vi "View A-Scan.vi"(10 "A-Scan Processed":sgl[](graph)=[-26.210978, -0.31578374, -1.8610598, -13.492583, -27.979498, -5.7245455, -0.3292389, -4.510563, -14.818077, -30.297182, -19.535238, -8.432641, -0.8121514, -1.7452242, -11.954155, -16.504982, -5.743655, -5.071388, -12.874917, -27.469084, -28.696384, -23.557272, -18.030994, -15.969668, -11.015175, -11.5916395, -19.863699, -26.249102, -22.386854, -29.339754, -25.127794, -33.261314, -28.425385, -31.03366, -23.45998, -24.344952, -31.405022, -32.837296, -28.08223, -25.55752, -25.279045, -26.942255, -26.625408, -24.167088, -27.910465, -29.274937, -22.219278, -20.05723, -26.108677, -22.097414, -27.75035, -32.056778, -29.910599, -24.903984, -27.671215, -29.608793, -44.94435, -32.444386, -36.56743, -24.9354, -26.683678, -23.9393, -25.238876, -35.807644, -28.46127, -33.92609, -23.394852, -20.960835, -19.181705, -18.781902, -22.780018, -31.818577, -28.909134, -22.674618, -25.622366, -31.60658, -29.545992, -34.63347, -27.351624, -45.00616, -30.52248, -34.17556, -26.224926, -28.119835, -25.108356, -32.589897, -21.198568, -21.048626, -24.815128, -20.277594, -22.449446, -22.564396, -23.654078, -19.366909, -25.552483, -17.816277, -18.52091, -25.534723, -25.30511, -21.510155, -21.73051, -23.231468, -23.07098, -25.038015, -21.5863, -38.30931, -27.069336, -29.471285, -23.319408, -23.01601, -24.3645, -32.88109, -23.353159, -25.882452, -28.715004, -34.466026, -34.025963, -35.122337, -22.841404, -22.532616, -12.578817, -11.619661, -17.050789, -25.473412, -30.49468, -31.098743, -41.366486, -28.964567, -38.44023, -26.351032, -21.317728, -21.813507, -23.792786, -20.529749, -20.11974, -23.277401, -27.823189, -26.973354, -24.241344, -24.333897, -26.06728, -53.132034, -32.367374, -31.709272, -29.559715, -35.48095, -40.987263, -30.28252, -28.209124, -29.503412, -27.401718, -27.646305, -22.93663, -22.070507, -33.09205, -34.82585, -27.275171, -32.58675, -29.522762, -22.635445, -23.142614, -27.973444, -26.65776, -27.490786, -39.08202, -23.444656, -22.362215, -22.415667, -33.80705, -28.281424, -26.454248, -37.24972, -43.585503, -27.439075, -27.784927, -27.602098, -32.125473, -35.726906, -36.536613, -31.075264, -38.49138, -27.625084, -26.77308, -27.488235, -29.514954, -22.231047, -29.748785, -33.403545, -27.761621, -26.688044, -25.825941, -35.921432, -43.165215, -26.127644, -26.853542, -24.654018, -22.703587, -27.379139, -35.317154, -24.985218, -20.411322, -22.853783, -30.926537, -30.707005, -31.797073, -31.337273, -26.2733, -23.047895, -22.52106, -27.7406, -27.451904, -33.804142, -27.606064, -25.81736, -27.720068, -36.016445, -27.700396, -27.664001, -30.901567, -27.07572, -32.00824, -26.91952, -23.52076, -23.271412, -25.111042, -34.587776, -32.977566, -25.886318, -24.229359, -26.734869, -32.142445, -26.288021, -30.677977, -52.17713, -24.04543, -22.249277, -34.459236, -30.383837, -32.543636, -32.750458, -26.37726, -23.7031, -27.623089, -32.123077, -40.254158, -23.576668, -24.094315, -30.320057, -31.964115, -29.275007, -33.622116, -30.901989, -25.8515, -22.568684, -24.535221, -25.86589, -37.747265, -31.16762, -36.97809, -34.62544, -29.410555, -25.7421, -24.113754, -24.21185, -26.27621, -28.80848, -33.13751, -29.363487, -31.258715, -24.950201, -27.174103, -22.409803, -22.727638, -30.952318, -31.949465, -33.96205, -32.321663, -41.727978, -26.914566, -23.141737, -22.170698, -20.978714, -27.677824, -24.802229, -20.999434, -25.072222, -28.95887, -32.70508, -28.58545, -27.07776, -24.924133, -25.208416, -28.979347, -25.955524, -32.08485, -28.693113, -29.154903, -37.858196, -39.133152, -36.21201, -25.883911, -23.183058, -25.838087, -26.123013, -29.354885, -27.11465, -24.470499, -27.968615, -23.639149, -23.14795, -26.119194, -35.968136, -28.441235, -23.77411, -23.665869, -31.111137, -31.179775, -28.989357, -27.464413, -32.31834, -26.286488, -27.108946, -29.648035, -27.614647, -36.93215, -32.280243, -29.210852, -25.338709, -27.051355, -25.309155, -23.086699, -31.160858, -28.991549, -27.485672, -27.540636, -21.71913, -26.28127, -31.117641, -23.571243, -22.516005, -29.04525, -32.098057, -25.547585, -42.95463, -31.956524, -22.141758, -17.952759, -19.610708, -23.644444, -27.758587, -25.057549, -26.134052, -25.293467, -29.953926, -29.844152, -23.126877, -26.776941, -33.989, -28.728153, -32.912956, -23.412436, -26.758936, -22.57225, -21.015762, -29.183378, -25.705784, -23.323528, -23.375137, -23.703573, -35.110134, -26.101551, -24.078419, -26.154135, -22.656559, -21.120544, -27.295572, -24.547276, -24.689686, -35.097187, -19.975447, -20.70405, -30.063946, -27.709393, -24.640957, -32.71785, -28.640612, -20.957756, -20.722157, -26.627188, -31.318886, -29.09002, -27.642347, -24.033022, -32.032455, -26.147396, -32.72879, -33.134163, -25.682604, -26.329826, -34.172707, -45.549637, -32.19201, -28.775599, -27.236197, -36.347317, -35.575523, -26.131685, -28.427603, -31.673988, -36.608932, -34.141914, -42.357056, -29.318504, -28.417885, -32.167183, -34.500694, -27.596508, -31.125277, -26.832617, -21.614109, -22.663319, -29.111574, -24.030752, -22.409107, -31.82102, -32.892212, -32.415745, -26.740353, -25.385103, -26.80175, -24.186478, -22.655315, -22.39489, -21.797451, -20.889229, -23.851068, -24.81073, -21.483337, -21.090714, -26.381187, -26.369854, -24.48166, -23.760208, -23.644342, -25.481583, -21.709759, -20.336998, -22.738392, -24.181318, -23.530704, -24.073698, -25.371855, -29.36827, -33.906986, -22.88837, -22.117483, -34.872936, -31.19501, -25.523607, -21.588385, -20.013102, -18.8254, -18.81281, -26.45252, -31.17826, -31.253874, -27.593842, -32.520233, -24.856508, -23.329897, -29.87441, -37.53676, -23.516674, -20.780876, -25.053402, -25.033222, -23.65327, -23.898222, -19.479591, -22.383928, -31.456697, -31.780369, -23.594852, -26.903454, -26.312883, -47.82139, -24.327026, -24.945843, -27.786072, -20.467207, -25.291618, -24.066692, -36.908745, -23.990826, -22.015648, -21.728424, -24.255674, -25.284016, -17.604519, -21.369007, -24.234962, -21.949186, -23.958088, -23.777592, -17.950075, -22.514679, -30.692993, -32.666252, -28.321722, -26.032763, -31.239384, -23.781271, -25.228098, -24.143929, -24.327179, -21.55861, -22.293808, -40.871967, -31.49052, -26.345123, -31.653671, -38.96815, -31.11382, -30.299416, -34.112003, -29.309956, -19.669268, -20.856876, -25.5818, -25.964798, -23.235428, -20.267351, -21.306042, -25.324953, -32.886566, -33.848198, -30.231703, -19.943031, -20.70887, -31.18996, -38.037865, -25.804028, -23.056585, -26.322596, -38.74378, -28.29768, -27.166054, -27.325365, -22.84835, -23.460272, -23.510675, -25.210625, -29.019207, -29.465004, -34.738686, -28.07248, -29.004747, -37.84001, -30.637262, -30.132875, -24.175072, -25.127258, -26.92854, -28.183363, -22.317673, -29.53536, -32.943462, -22.5015, -17.434628, -17.622349, -21.835793, -21.983576, -21.254726, -24.232197, -30.984581, -35.853207, -32.10312, -19.321465, -17.624142, -20.444664, -21.004726, -22.67358, -25.06542, -21.320122, -23.435019, -27.823555, -26.044563, -24.597794, -22.637848, -24.535957, -34.368435, -24.400473, -20.907734, -25.545467, -35.642853, -26.396896, -25.6619, -25.823061, -20.670412, -20.21106, -29.578287, -29.226358, -30.222311, -27.00819, -28.136663, -29.100351, -28.457932, -24.669703, -25.028812, -18.786524, -19.427868, -25.43777, -21.199684, -15.573761, -1.0208147, 7.6145773, 10.022359, 7.7157907, 6.070616, 9.813012, 15.933785, 22.136951, 25.04485, 23.8101, 16.993906, 3.8796186, 15.961233, 16.285875, 13.045634, 7.2316785, 2.657391, -4.7237477, -6.347074, -5.0806813, -11.554905, -26.610163, -9.1125765, -11.753917, -10.766447, -12.167433, -17.402613, -9.076464, -10.4888525, -20.842134, -13.619364, -16.773762, -19.546986, -23.723976, -25.914572, -28.425293, -18.009684, -15.721116, -19.651096, -22.298372, -26.993717, -21.207827, -33.86458, -16.998291, -19.768642, -22.319141, -18.725727, -20.68567, -23.248938, -33.058094, -35.201458, -30.761806, -26.134024, -40.351723, -17.83051, -14.775904, -20.180481, -26.82964, -22.300451, -23.828773, -22.818367, -23.048168, -26.578943, -26.982422, -30.778564, -32.837204, -29.521778, -31.278343, -35.43119, -36.43036, -31.21062, -26.882355, -25.316109, -30.444912], 11 "A-Scan (Raw)":u16[](graph)=[33360, 31728, 32832, 32768, 32272, 32560, 32976, 32608, 33136, 31744, 33296, 31472, 32848, 33264, 31968, 33120, 32272, 32608, 32944, 32112, 33456, 32016, 33584, 31952, 33488, 31552, 33632, 33344, 33360, 32128, 32368, 33232, 31824, 33280, 31632, 34576, 31136, 33456, 31360, 33344, 32208, 32848, 32800, 31920, 34288, 31168, 33520, 31408, 33488, 31760, 33264, 32544, 32352, 33280, 31904, 33696, 31808, 33776, 32256, 33456, 32096, 32864, 32800, 32304, 33408, 31952, 33840, 31568, 33584, 31888, 33424, 32448, 32592, 33008, 32032, 33584, 31856, 33872, 32112, 33328, 32096, 32704, 32752, 32368, 33632, 32176, 33456, 31776, 33456, 31952, 33184, 32256, 32640, 32848, 32096, 33408, 31808, 33552, 32464, 34304, 31952, 32800, 32576, 32224, 33216, 32144, 33472, 31936, 33920, 31920, 33168, 33216, 32448, 32800, 32128, 33424, 31760, 33408, 31904, 33328, 32208, 32960, 32912, 32368, 33104, 32016, 33328, 31808, 33856, 31888, 33248, 32592, 32928, 32896, 32464, 33456, 32464, 33232, 31968, 33264, 32160, 33120, 32672, 33008, 32864, 32208, 33232, 31968, 33264, 31744, 33200, 32160, 32864, 32752, 32496, 33280, 32256, 33408, 32176, 33488, 32096, 32976, 32320, 32720, 32976, 32288, 33232, 31888, 33568, 31776, 33408, 32096, 32976, 32480, 32656, 33168, 32240, 33408, 31936, 33552, 32048, 33312, 32080, 32768, 32736, 32320, 33328, 32128, 33632, 31872, 33584, 31632, 33296, 32048, 32688, 32912, 32224, 33392, 31600, 33920, 31600, 33952, 31728, 33264, 32304, 32512, 33008, 31872, 33840, 31408, 34176, 31520, 33936, 31776, 33376, 32576, 32240, 33376, 31440, 34064, 31136, 34416, 31280, 34016, 31936, 33232, 32928, 32096, 33584, 31200, 34288, 30864, 34384, 31280, 33952, 32000, 32800, 33088, 31600, 33936, 30752, 34480, 30608, 34304, 31216, 33504, 32256, 32464, 33456, 31120, 34352, 30464, 34704, 30448, 34496, 31232, 33488, 32480, 32144, 33952, 30944, 34608, 30432, 34736, 30752, 34176, 31760, 33152, 33232, 31872, 34368, 30672, 35056, 30480, 34656, 30976, 33840, 32352, 32512, 33808, 31184, 34912, 30496, 35056, 30512, 34432, 31520, 33248, 32864, 31744, 34224, 30736, 35184, 30240, 34928, 30704, 33968, 31952, 32624, 33744, 31152, 34848, 30480, 35344, 30416, 34816, 31216, 33488, 32640, 32048, 34000, 30800, 35040, 30304, 35280, 30704, 34560, 31872, 32992, 33232, 31632, 34400, 30560, 35280, 30352, 35088, 31120, 33888, 32544, 32608, 33696, 31248, 34832, 30576, 35152, 30640, 34800, 31376, 33552, 32784, 32208, 33952, 30992, 34608, 30608, 34704, 30864, 34064, 31888, 32992, 33264, 31632, 34080, 30752, 34416, 30608, 34144, 31312, 33568, 32432, 32144, 33488, 31328, 34160, 30752, 34272, 30880, 33904, 31744, 32960, 32912, 31984, 33776, 31184, 34192, 31008, 34016, 31360, 33456, 32096, 32752, 33328, 31776, 34096, 31312, 34160, 31296, 33872, 31840, 33152, 32688, 32176, 33696, 31600, 34208, 31408, 34112, 31504, 33520, 32208, 32848, 32880, 31904, 33792, 31440, 34096, 31456, 33952, 31776, 33296, 32496, 32464, 33200, 31664, 33888, 31152, 34080, 31344, 33808, 31904, 33024, 32768, 32096, 33488, 31328, 34016, 31104, 34096, 31408, 33712, 32160, 32640, 33120, 31744, 33744, 31264, 34176, 30992, 34000, 31600, 33296, 32560, 32384, 33440, 31344, 34096, 31056, 34272, 31136, 34000, 31888, 33056, 32880, 31888, 34016, 30992, 34480, 30560, 34448, 30976, 33648, 32224, 32448, 33456, 31312, 34336, 30432, 34800, 30240, 34528, 31040, 33376, 32432, 31776, 34048, 30528, 35088, 29744, 35376, 29936, 34672, 31072, 33152, 33168, 31200, 34624, 29968, 35760, 29344, 35600, 29904, 34336, 31520, 32720, 33472, 30896, 35312, 29472, 36144, 29344, 35536, 30320, 34240, 32048, 32144, 34496, 30144, 35984, 29152, 36432, 29392, 35456, 30864, 33664, 33008, 31200, 35056, 29648, 36464, 28912, 36368, 29648, 35216, 31408, 32864, 34000, 30336, 35824, 28832, 36672, 28784, 36304, 29968, 34576, 32336, 31712, 34800, 29776, 36512, 28592, 36848, 29104, 35808, 30608, 33808, 33296, 31264, 35344, 29136, 36752, 28688, 36752, 29376, 35472, 31344, 33008, 34128, 30544, 36032, 28976, 36848, 28816, 36528, 30112, 34720, 32080, 32496, 34512, 30112, 36288, 28640, 36880, 28880, 35792, 30448, 34048, 32704, 31728, 34960, 29728, 36336, 28880, 36544, 29152, 35344, 31248, 33360, 33248, 30960, 35088, 29488, 36128, 29024, 36048, 29824, 34672, 31632, 32800, 33520, 30800, 35312, 29504, 35968, 29264, 35552, 30272, 34288, 32080, 32288, 33920, 30752, 35344, 29696, 35744, 29840, 35120, 30896, 33808, 32576, 32256, 34208, 30928, 35088, 30192, 35440, 30384, 34800, 31328, 33712, 32784, 31984, 34208, 30880, 35008, 30496, 35168, 30768, 34544, 31680, 33200, 32976, 31984, 34048, 31120, 34784, 30816, 34720, 31216, 33984, 32096, 32976, 33136, 31888, 34064, 31152, 34640, 31024, 34496, 31264, 33920, 32256, 32688, 33296, 31728, 34128, 31264, 34384, 31120, 34208, 31488, 33488, 32368, 32528, 33248, 31584, 33888, 31168, 34192, 31200, 33936, 31616, 33248, 32416, 32256, 33296, 31376, 34016, 30992, 34096, 31168, 33648, 31680, 33088, 32608, 31952, 33312, 31392, 33888, 31136, 33888, 31296, 33392, 32048, 32656, 32912, 31808, 33488, 31248, 33904, 31328, 33648, 31728, 33168, 32528, 32336, 33440, 31584, 33936, 31408, 34112, 31568, 33680, 32368, 33024, 33120, 32176, 33712, 31648, 34176, 31536, 33936, 31952, 33328, 32768, 32576, 33504, 32016, 34256, 31552, 34304, 31664, 33824, 32368, 33120, 33232, 32336, 34064, 31568, 34480, 31504, 34208, 31968, 33584, 32640, 32656, 33648, 31776, 34352, 31312, 34528, 31424, 34144, 32064, 33328, 33328, 32144, 34160, 31344, 34608, 31184, 34512, 31408, 33936, 32416, 32928, 33456, 31952, 34368, 31216, 34736, 31184, 34528, 31696, 33648, 33008, 32512, 33904, 31488, 34624, 30960, 34768, 31200, 34400, 31872, 33120, 33104, 31952, 34240, 31024, 34928, 30752, 34848, 31136, 34256, 32240, 32928, 33360, 31824, 34432, 30928, 35056, 30656, 34992, 31200, 34144, 32224, 32768, 33824, 31424, 34816, 30656, 35232, 30608, 34944, 31232, 33936, 32608, 32672, 33904, 31264, 34928, 30496, 35296, 30512, 34960, 31280, 33936, 32480, 32624, 33872, 31344, 34976, 30528, 35312, 30544, 34928, 31216, 33920, 32512, 32496, 33952, 31184, 34976, 30496, 35168, 30560, 34944, 31200, 33712, 32864, 32304, 34080, 31248, 35040, 30512, 35328, 30736, 34880, 31312, 33776, 32784, 32512, 33824, 31216, 35024, 30560, 35344, 30576, 34880, 31232, 33872, 32592, 32544, 34144, 31232, 35040, 30592, 35200, 30640, 34688, 31392, 33504, 32816, 32256, 33968, 31344, 34896, 30624, 35136, 30816, 34512, 31648, 33568, 32672, 32352, 33824, 30960, 34704, 30512, 34960, 30736, 34528, 31488, 33216, 32448, 32048, 33808, 30912, 34528, 30432, 34752, 30672, 34224, 31376, 33344, 32544, 32272, 33648, 31008, 34192, 30608, 34400, 30816, 33920, 31488, 33184, 32544, 32096, 33536, 31376, 34128, 30992, 34176, 31280, 33744, 31984, 32944, 32768, 32272, 33616, 31696, 34080, 31600, 34096, 31824, 33824, 32400, 32928, 33056, 32240, 33600, 31872, 34032, 31872, 34096, 32144, 33680, 32752, 33088, 33344, 32544, 33712, 32208, 33984, 32064, 33904, 32656, 33456, 33072, 32992, 33552, 32608, 33824, 32464, 34000, 32336, 33632, 32752, 33312, 33104, 32832, 33552, 32528, 33840, 32336, 33776, 32272, 33648, 32784, 33152, 32976, 32656, 33456, 32304, 33488, 32256, 33568, 32352, 33440, 32864, 32976, 33120, 32544, 33376, 32208, 33392, 32112, 33376, 32320, 32944, 32656, 32736, 32960, 32352, 33232, 32320, 33328, 32272, 33200, 32400, 32912, 32704, 32544, 33088, 32144, 33328, 32160, 33312, 32352, 33088, 32688, 32848, 33168, 32416, 33424, 32176, 33568, 32112, 33296, 32384, 33040, 32880, 32640, 33344, 32368, 33744, 32192, 33904, 32288, 33600, 32720, 33184, 32832, 32640, 33392, 32160, 33872, 31952, 34016, 32080, 33776, 32768, 33232, 33104, 32688, 33520, 31952, 33872, 31744, 33824, 31952, 33456, 32336, 33008, 33008, 32432, 33648, 31760, 34032, 31616, 33888, 31872, 33344, 32176, 32800, 32912, 32112, 33552, 31520, 33968, 31376, 33872, 31808, 33488, 32368, 32640, 32928, 31952, 33456, 31312, 33952, 31024, 33760, 31520, 33264, 32240, 32512, 33120, 31856, 33776, 31136, 34112, 31056, 33888, 31584, 33248, 32304, 32432, 33104, 31728, 33856, 31008, 34352, 31136, 34176, 31504, 33632, 32336, 32512, 33152, 31632, 33872, 30992, 34256, 31024, 34144, 31360, 33600, 32336, 32800, 33312, 31872, 33968, 31088, 34304, 31136, 34192, 31408, 33712, 32256, 32656, 33184, 31872, 33952, 31312, 34240, 31104, 34176, 31536, 33472, 32096, 32496, 32992, 31808, 33568, 31376, 34016, 31136, 34144, 31536, 33536, 32304, 32880, 33152, 32128, 33648, 31600, 33888, 31360, 33776, 31760, 33264, 32304, 32592, 33136, 32080, 33792, 31744, 33968, 31696, 33920, 32032, 33456, 32576, 32736, 33120, 32144, 33616, 31744, 33856, 31808, 33792, 32064, 33552, 32800, 32992, 33200, 32432, 33616, 31936, 33776, 31936, 33680, 32096, 33280, 32752, 32816, 33312, 32512, 33616, 32224, 33648, 32224, 33488, 32432, 33056, 32768, 32624, 33184, 32256, 33536, 32000, 33648, 32064, 33360, 32352, 33024, 32800, 32688, 33056, 32224, 33376, 31824, 33568, 31952, 33280, 32240, 32864, 32688, 32544, 33088, 32208, 33248, 31984, 33392, 31904, 33232, 32080, 32784, 32624, 32448, 32752, 32256, 33152, 32048, 33344, 31984, 33328, 32304, 32960, 32848, 32656, 32944, 32256, 33136, 32208, 33296, 32128, 33104, 32352, 32832, 32672, 32656, 33168, 32464, 33312, 32528, 33264, 32576, 33184, 32576, 32832, 32848, 32608, 33152, 32368, 33168, 32512, 33040, 32784, 33040, 32992, 32800, 33008, 32512, 33248, 32224, 33312, 32464, 33120, 32688, 32800, 32960, 32528, 33104, 32448, 33248, 32304, 33296, 32368, 33072, 32880, 32592, 33328, 32208, 33296, 32176, 33136, 32032, 33184, 32160, 32880, 32720, 32432, 33008, 31920, 33328, 31952, 33360, 31888, 33168, 31968, 32800, 32304, 32144, 32976, 31552, 33168, 31328, 33200, 31728, 32912, 32064, 32848, 32464, 32448, 33120, 31904, 33344, 31568, 33360, 31712, 33008, 32128, 32608, 32816]) -> ()   [LabVIEW 2015, in "Processing.lvclass"]
uses:
  Processing.lvclass
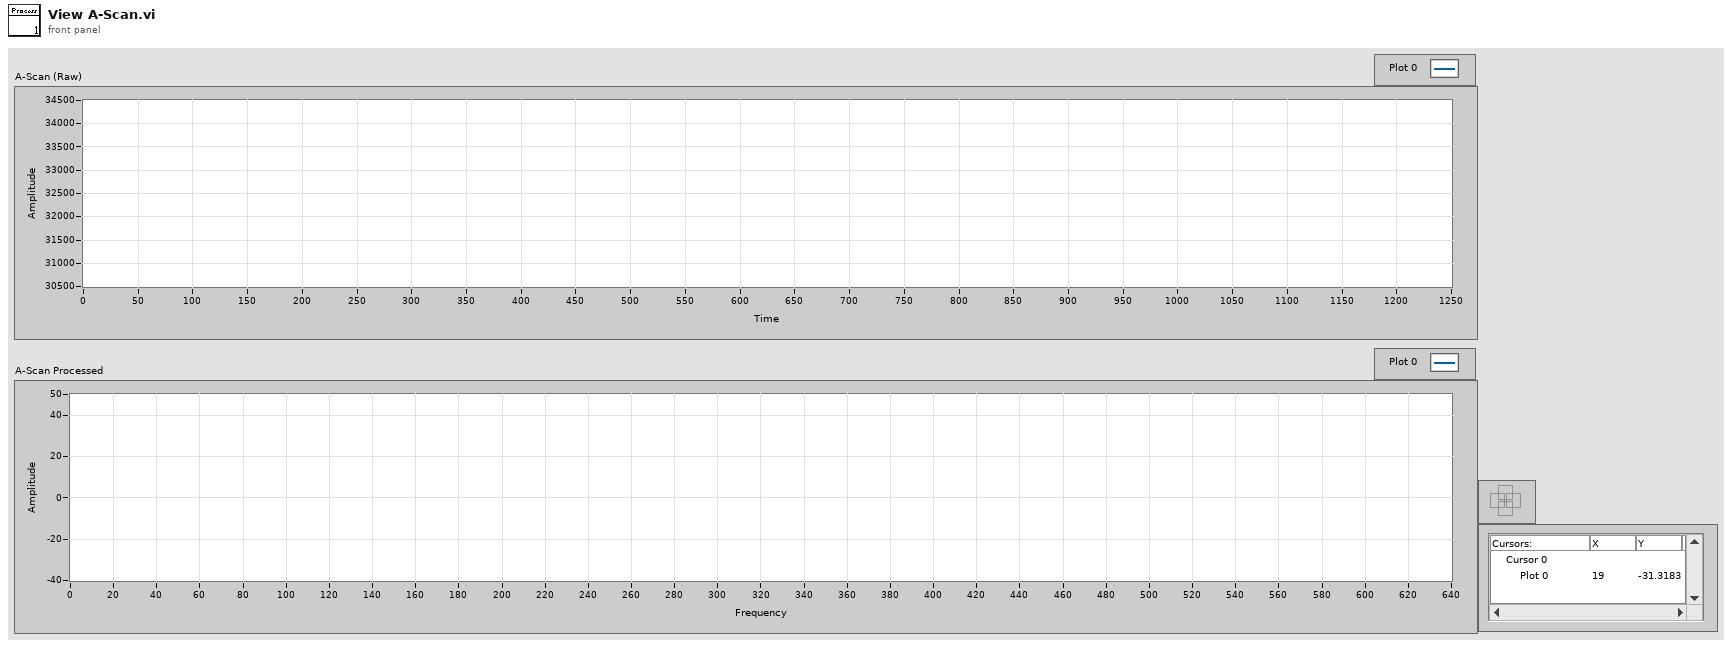
[diagram p1: front panel]
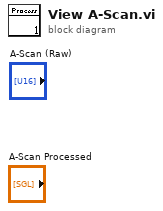
[diagram p0: block diagram]
diagram:
